vi "ListParam.vi"(0 "Start AC RMS Volt":i32, 1 "End AC RMS Volt":i32, 2 "Time/Cycles":i32, 3 "Start DC Volt":i32, 4 "End DC RMS Volt":i32, 5 "Start Freq":i32, 6 "End Freq":i32, 7 "Steps":i32) -> (8 "List Write paramters":string)   [LabVIEW 2018, in "BK Precision 983X Series.lvlib"]
uses:
  <instrlib>/BK Precision 983X Series/BK Precision 983X Series.lvlib
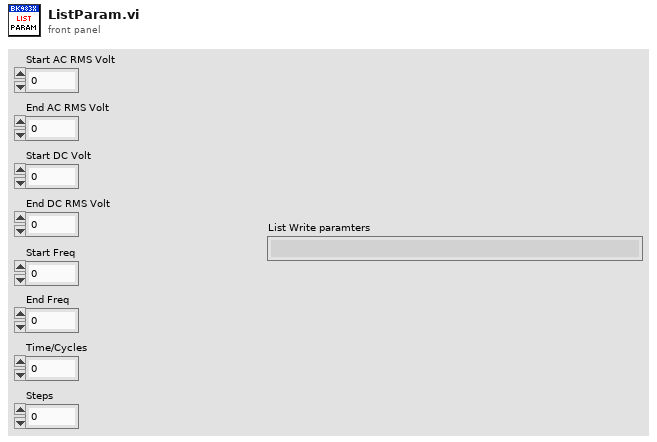
[diagram p1: front panel]
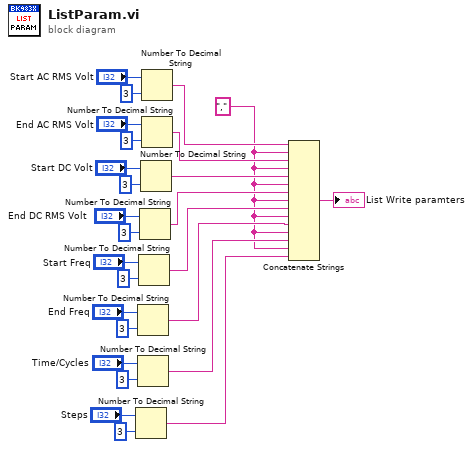
[diagram p0: block diagram]
diagram:
  w1 = ","
  n1 = Number To Decimal String(number="Steps", width (-)=i16 3) -> (decimal integer string=w2:string)
  n2 = Number To Decimal String(number="End Freq", width (-)=i16 3) -> (decimal integer string=w7:string)
  n3 = Number To Decimal String(number="Time/Cycles", width (-)=i16 3) -> (decimal integer string=w6:string)
  n4 = Number To Decimal String(number="Start Freq", width (-)=i16 3) -> (decimal integer string=w8:string)
  n5 = Number To Decimal String(number="End DC RMS Volt", width (-)=i16 3) -> (decimal integer string=w9:string)
  n6 = Number To Decimal String(number="Start DC Volt", width (-)=i16 3) -> (decimal integer string=w10:string)
  n7 = Number To Decimal String(number="Start AC RMS Volt", width (-)=i16 3) -> (decimal integer string=w26:string)
  n8 = Number To Decimal String(number="End AC RMS Volt", width (-)=i16 3) -> (decimal integer string=w11:string)
  n9 = Concatenate Strings(w26, w1, w11, w1, w10, w1, w9, w1, w8, w1, w7, w1, w6, w1, w2) -> (→"List Write paramters":string)
